vi "Handle UNREGISTERED.vi"(8 "error in (no error)":errorcluster, 9 "WAMP Message":T15, 10 "Message loop data (in)":T1, 11 "reference":refnum<class "WAMP Client.lvclass">) -> (0 "error out":errorcluster, 2 "Message Loop Data (Out)":T1, 3 "reference out":refnum<class "WAMP Client.lvclass">)   [LabVIEW 2020, in "wamplv.lvlib" / "WAMP Client.lvclass"]
uses:
  WAMP Client.lvclass
  WAMP Client.lvclass/WAMP Client.ctl
  API/TypeDefs/WAMP error.ctl
  API/TypeDefs/Combined error.ctl
  TypeDef/Success or error.ctl
  270ddf32-b247-4482-b6bc-5475b82892bf.vi
  TypeDef/EVENT payload.ctl
  TypeDef/Subscription Details.ctl
  Private/TypeDefs/WAMP Message Codes.ctl
  wamplv.lvlib
  TypeDef/WAMP Received Message.ctl
  TypeDef/UNSUBSCRIBE Result.ctl
  TypeDef/UNSUBSCRIBE Request Data.ctl
  TypeDef/Unsubscribe Requests Map.ctl
  TypeDef/REGISTER Request Data.ctl
  TypeDef/PUBLISH Request Data.ctl
  TypeDef/Publish Requests Map.ctl
  TypeDef/Endpoint Data.ctl
  TypeDef/CALL Request Map.ctl
  TypeDef/Subscribe Result.ctl
  TypeDef/SUBSCRIBE Request Data.ctl
  TypeDef/SUBSCRIBE Requests Map.ctl
  TypeDef/Subscriptions Map.ctl
  TypeDef/Message Loop Data.ctl
  TypeDef/Unregister request.ctl
  TypeDef/Unregister requests map.ctl
  TypeDef/PUBLISH result.ctl
  Private/Requests/Call/ICallRequest/ICallRequest.lvclass
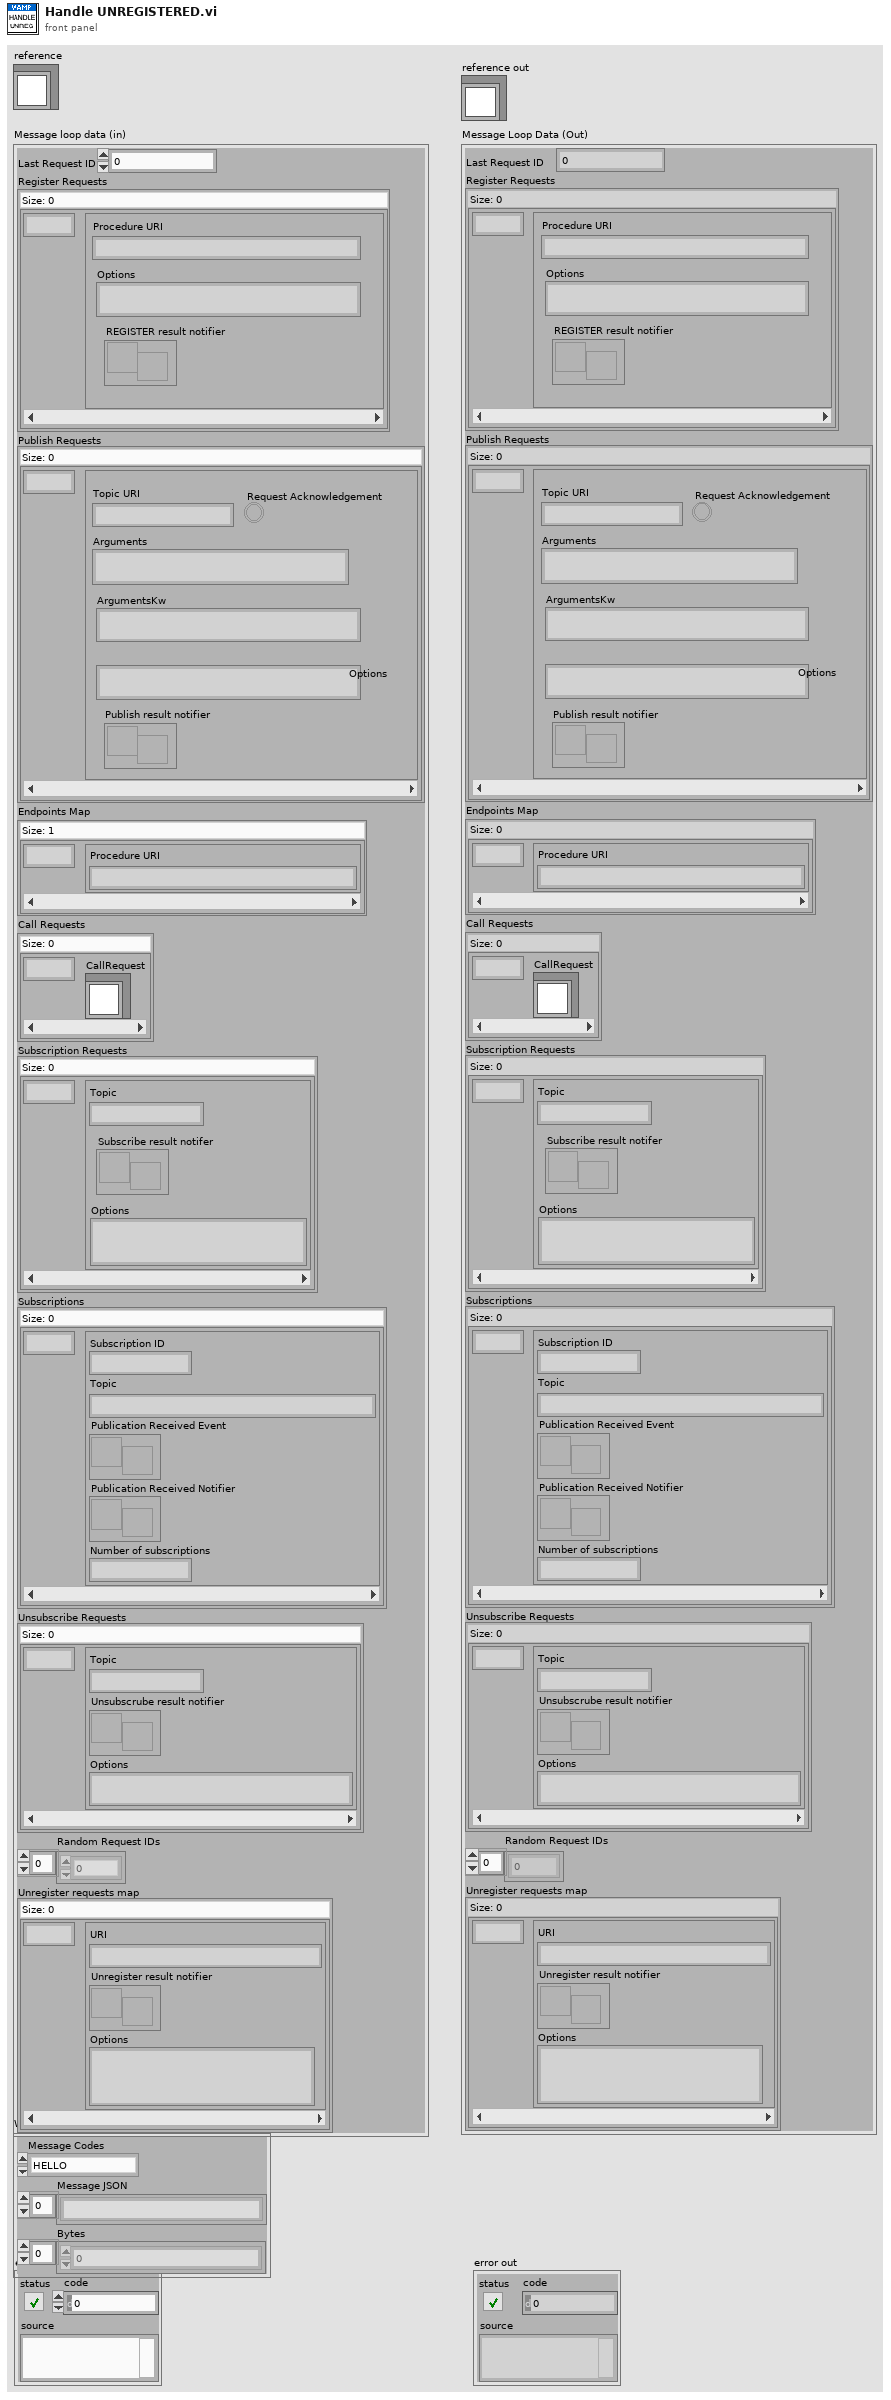
[diagram p1: front panel]
types:
  T1 = typedef "wamplv.lvlib/WAMP Client.lvclass/Message Loop Data.ctl" = cluster{"Last Request ID":u64, "Register Requests":map{u64, T2}, "Publish Requests":T3, "Endpoints Map":map{u64, T5}, "Call Requests":T6, "Subscription Requests":T7, "Subscriptions":T9, "Unsubscribe Requests":T11, "Random Request IDs":u64[], "Unregister requests map":T13}
  T2 = typedef "wamplv.lvlib/WAMP Client.lvclass/REGISTER Request Data.ctl" = cluster{"Procedure URI":string, "Options":string, "REGISTER result notifier":refnum<notifier>}
  T3 = typedef "wamplv.lvlib/WAMP Client.lvclass/Publish Requests Map.ctl" = map{u64, T4}
  T4 = typedef "wamplv.lvlib/WAMP Client.lvclass/PUBLISH Request Data.ctl" = cluster{"Topic URI":string, "Arguments":string, "ArgumentsKw":string, "Request Acknowledgement":bool, "Options":string, "Publish result notifier":refnum<notifier>}
  T5 = typedef "wamplv.lvlib/WAMP Client.lvclass/Endpoint Data.ctl" = cluster{"Procedure URI":string}
  T6 = typedef "wamplv.lvlib/WAMP Client.lvclass/CALL Request Map.ctl" = map{u64, refnum<class "ICallRequest.lvclass">}
  T7 = typedef "wamplv.lvlib/WAMP Client.lvclass/SUBSCRIBE Requests Map.ctl" = map{u64, T8}
  T8 = typedef "wamplv.lvlib/WAMP Client.lvclass/SUBSCRIBE Request Data.ctl" = cluster{"Topic":string, "Subscribe result notifer":refnum<notifier>, "Options":string}
  T9 = typedef "wamplv.lvlib/WAMP Client.lvclass/Subscriptions Map.ctl" = map{u64, T10}
  T10 = typedef "wamplv.lvlib/WAMP Client.lvclass/Subscription Details.ctl" = cluster{"Subscription ID":u64, "Topic":string, "Publication Received Event":refnum<user-event>, "Publication Received Notifier":refnum<notifier>, "Number of subscriptions":u64}
  T11 = typedef "wamplv.lvlib/WAMP Client.lvclass/Unsubscribe Requests Map.ctl" = map{u64, T12}
  T12 = typedef "wamplv.lvlib/WAMP Client.lvclass/UNSUBSCRIBE Request Data.ctl" = cluster{"Topic":string, "Unsubscrube result notifier":refnum<notifier>, "Options":string}
  T13 = typedef "wamplv.lvlib/WAMP Client.lvclass/Unregister requests map.ctl" = map{u64, T14}
  T14 = typedef "wamplv.lvlib/WAMP Client.lvclass/Unregister request.ctl" = cluster{"URI":string, "Unregister result notifier":refnum<notifier>, "Options":string}
  T15 = typedef "wamplv.lvlib/WAMP Client.lvclass/WAMP Received Message.ctl" = cluster{"Message Codes":T16, "Message JSON":string[], "Bytes":u8[]}
  T16 = typedef "wamplv.lvlib/WAMP Message Codes.ctl" = enum8{"HELLO", "WELCOME", "ABORT", "GOODBYE", "ERROR", "PUBLISH", "PUBLISHED", "SUBSCRIBE", "SUBSCRIBED", "UNSUBSCRIBE", "UNSUBSCRIBED", "EVENT", "CALL", "RESULT", "REGISTER", "REGISTERED", "UNREGISTER", "UNREGISTERED", "INVOCATION", "YIELD"}
  T17 = typedef "wamplv.lvlib/WAMP Client.lvclass/Success or error.ctl" = cluster{"Success?":bool, "URI":string, "Combined Error":T18}
  T18 = typedef "wamplv.lvlib/WAMP Client.lvclass/Combined error.ctl" = cluster{"Error?":bool, "WAMP Error":T19, "Error":errorcluster}
  T19 = typedef "wamplv.lvlib/WAMP Client.lvclass/WAMP error.ctl" = cluster{"Details":string, "ArgumentKw Payload":string, "Error?":bool, "Error URI":string, "Arguments Payload":string}
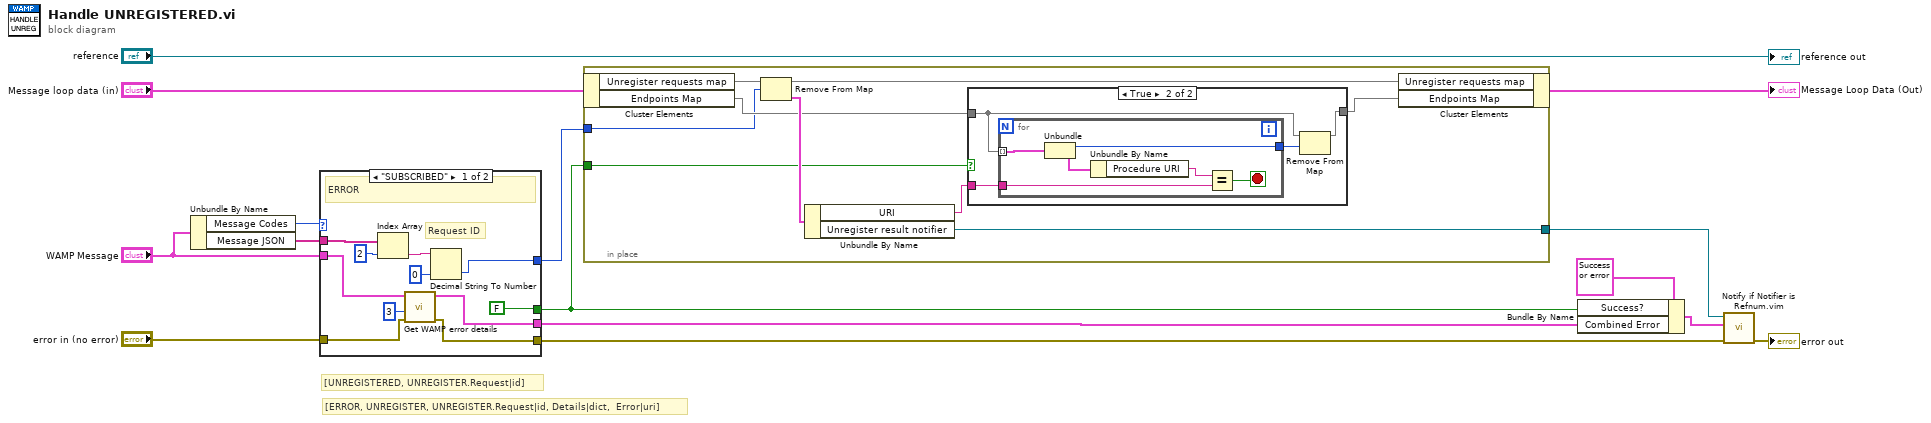
[diagram p0: block diagram]
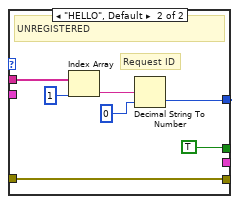
[diagram p3: hidden frame]
diagram:
  # "[UNREGISTERED, UNREGISTER.Request|id]"
  # "[ERROR, UNREGISTER, UNREGISTER.Request|id, Details|dict,  Error|uri]"
  n1 = Unbundle By Name("WAMP Message") -> ("Message Codes"=w12:T16, "Message JSON"=w11:string[])
  n2 = case shown="\"SUBSCRIBED\"" w12 {
    tunnel: w11 -> [w24 w32]
    tunnel: [w23 w27] -> w3
    tunnel: "error in (no error)" -> [w16 w31]
    tunnel: [w17 w31] -> w7
    tunnel: [w18 _] -> w14
    tunnel: [FALSE ("Success?") TRUE ("Success?")] -> w2
    tunnel: "WAMP Message" -> [w20 _]
    frame "SUBSCRIBED" {
      # "Request ID"
      # "ERROR"
      n3 = Index Array(array=w24, index=2) -> (element=w25:string)
      n4 = call "Get WAMP error details.vi"("error in (no error)"=w16, "Details Index"=u32 3, "WAMP Message"=w20) -> ("error out"=w17:errorcluster, "Combined Error"=w18:T18)  [unwired: 6 in, 1 out]
      n5 = Decimal String To Number(string=w25, default (0L)=u64 0 ("default (0 I32)")) -> (number=w23:u64)  [unwired: 1 in, 1 out]
    }
    frame "HELLO", Default {
      # "Request ID"
      # "UNREGISTERED"
      n6 = Index Array(array=w32, index=1) -> (element=w29:string)
      n7 = Decimal String To Number(string=w29, default (0L)=u64 0) -> (number=w27:u64)  [unwired: 1 in, 1 out]
    }
  }
  n8 = in-place {
    in-place-border: [w36] -> w5
    in-place-border: w3 -> [w35]
    in-place-border: w2 -> [w34]
    n9 = in-place-cluster #1("Message loop data (in)") -> ("Unregister requests map"=w42:T13, "Endpoints Map"=w38:map{u64, T5})
    n10 = Remove From Map(10:w35, 11:w42) -> (1:w40:T14, 3:w41:T13)  [unwired: 1 out]
    n11 = Unbundle By Name(w40) -> ("URI"=w39:string, "Unregister result notifier"=w36:refnum<notifier>)
    n12 = case shown="True" w34 {
      tunnel: w39 -> [_ w47]
      tunnel: w38 -> [w43 w45]
      tunnel: [w43 w44] -> w37
      frame False {
      }
      frame True {
        n13 = for {
          tunnel: [w51] -> w46
          tunnel: w45 -> [w49] mode=indexing
          tunnel: w47 -> [w48]
          stop <- w52 stop-if-true
          n14 = Unbundle(w49) -> ("key"=w51:u64, "Endpoint Data"=w53:T5)
          n15 = Unbundle By Name(w53) -> ("Procedure URI"=w50:string)
          n16 = Equal?(x=w50, y=w48) -> (x = y?=w52:bool)
        }
        n17 = Remove From Map(10:w46, 11:w45) -> (3:w44:map{u64, T5})  [unwired: 2 out]
      }
    }
    n18 = in-place-cluster #1("Unregister requests map"=w41, "Endpoints Map"=w37) -> (→"Message Loop Data (Out)":T1)
  }
  n19 = Bundle By Name(cluster=T17 {"Success?"=FALSE, "URI"="", "Combined Error"={"Error?"=FALSE, "WAMP Error"={"Details"="{}", "ArgumentKw Payload"="{}", "Error?"=FALSE, "Error URI"="", "Arguments Payload"=""}, "Error"={"status"=FALSE, "code"=0, "source"=""}}} ("Sucess or error"), "Success?"=w2, "Combined Error"=w14) -> (w6:T17)
  n20 = call "Notify if Notifier is Refnum.vim"("error in (no error)"=w7, "RESULT Payload"=w6, "Notifier in"=w5) -> ("error out"=→"error out":errorcluster)  [unwired: 8 in]
  "reference out" <- "reference"
